vi "游戏提示框.vi"(0 "数值1":dbl, 2 "再来一局可见":bool, 3 "结果":string, 5 "数值2":dbl, 9 "数值3":dbl, 11 "数值4":dbl, 12 "返回游戏可见":bool, 13 "答案":string) -> (1 "指示灯 2":bool, 4 "扑克牌 1":u16(ring), 6 "扑克牌 2":u16(ring), 10 "扑克牌 3":u16(ring), 14 "指示灯":bool, 15 "扑克牌 4":u16(ring))   [LabVIEW 2014]
panel:
  in  "再来一局":bool
  in  "返回游戏":bool
  out "正确答案：":string
  in  "退出游戏":bool
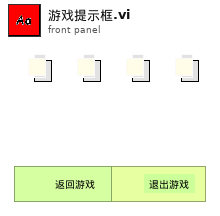
[diagram p1: front panel]
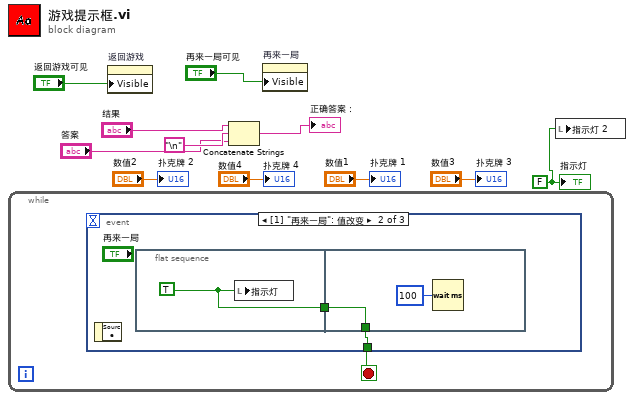
[diagram p0: block diagram]
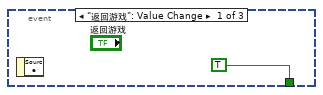
[diagram p2: hidden frame]
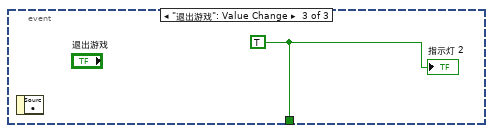
[diagram p3: hidden frame]
diagram:
  w3 = FALSE ("指示灯")
  n1 = while {
    stop <- w12 stop-if-true
    n2 = event shown="[1] \"再来一局\": 值改变" {
      selector: _ -> [_ _ _]
      dyn-events: _ -> [_ _ _]
      timeout: _ -> [_ _ _]
      tunnel: [TRUE w15 w19] -> w12
      event "返回游戏": Value Change {
        n3 = event-data() -> ()  [unwired: 1 in, 1 out]
      }
      event "再来一局": Value Change {
        n4 = event-data() -> ()  [unwired: 1 in, 1 out]
        n5 = flat-sequence {
          tunnel: [w16] -> w14
          tunnel: [w17] -> w15
          tunnel: w14 -> [w17]
          frame #0 {
            w16 = TRUE
            n6 = local write "指示灯"(w16) -> ()
          }
          frame #1 {
            n7 = Wait (ms)(milliseconds to wait=u32 100 ("等待时间（毫秒）")) -> ()  [unwired: 1 out]
          }
        }
      }
      event "退出游戏": Value Change {
        w19 = TRUE ("退出？(T)")
        n8 = event-data() -> ()  [unwired: 1 in, 1 out]
        "指示灯 2" <- w19
      }
    }
  }
  n9 = property on="返回游戏" class="Bool"("Visible"="返回游戏可见") -> ()  [unwired: 2 in, 2 out]
  n10 = Concatenate Strings("结果", "\n", "答案") -> (→"正确答案：":string)
  n11 = property on="再来一局" class="Bool"("Visible"="再来一局可见") -> ()  [unwired: 2 in, 2 out]
  n12 = local write "指示灯 2"(w3) -> ()
  "指示灯" <- w3
  "扑克牌 1" <- "数值1"
  "扑克牌 2" <- "数值2"
  "扑克牌 3" <- "数值3"
  "扑克牌 4" <- "数值4"
